vi "Process.vi"(0 "reference in":refnum<class "DCIR_HPPC.lvclass">, 5 "error in":errorcluster) -> (14 "reference out":refnum<class "DCIR_HPPC.lvclass">, 19 "error out":errorcluster)   [LabVIEW 2023, in "DCIR_HPPC.lvclass"]
uses:
  DCIR_HPPC.lvclass
  HPPC Parameters.ctl
  HPPC Mode.ctl
  Logger_class/Logger.lvclass
  builds/PowerModuleInterface/PowerModuleInterface.lvlibp/Classes/PowerModule_interface/PowerModuleInterface.lvclass
  <vilib>/Utility/NIReport.llb/Report Type.ctl
  <vilib>/printing/OpenHTMLReport.llb/Open HTML Report in Browser (Refnum).vi
  <vilib>/Utility/NIReport.llb/NI_report.lvclass
  DCIR_HPPC.lvclass/DCIR_HPPC.ctl
  <vilib>/Utility/SystemLogging/NI_SystemLogging.lvlib
  <userlib>/_OpenG.lib/time/time.llb/openg_time.lvlib
  <vilib>/Utility/NIReport.llb/NI_ReportGenerationCore.lvlib
panel:
  out "Last Command":string
  out "error info":errorcluster
  in  "Save HPPC Report":bool
  in  "HPPC Tab Control":T1(tab)
  out "HPPC Parameters":T2={"HPPC Mode"=1, "Pulse Duration (S)"=500.0, "Charge Current (A)"=1000.0, "Rest Duration (S)"=2.0, "Discharge Current (A)"=10.0, "Temperature (C)"=25.0, "Nominal Capacity (Ah)"=10.0, "Initial SoC (%)"=650.0, "Final SoC (%)"=50.0, "SoC Interval (%)"=10.0, "SoC Step Current (A)"=10.0, "SoC Step Relax (S)"=10.0} {"HPPC Mode" items=["One Shot (DCIR)", "Discharge Only", "Full Cycle"]; "Nominal Capacity (Ah)" min=0.0 max=100.0; "Final SoC (%)" min=0.0 max=100.0; "SoC Interval (%)" min=0.0 max=100.0; "Initial SoC (%)" min=0.0 max=100.0}
  out "HPPC Profile":waveform(dbl)[](graph)
  out "Running Status Log":i32(listbox) caption="TEST SERVER LOG"
  out "HPPC Step":dbl[][](graph)
  out "HPPC Voltage":cluster{dbl[], dbl[]}(graph)
  out "HPPC Power":cluster{dbl[], dbl[]}(graph)
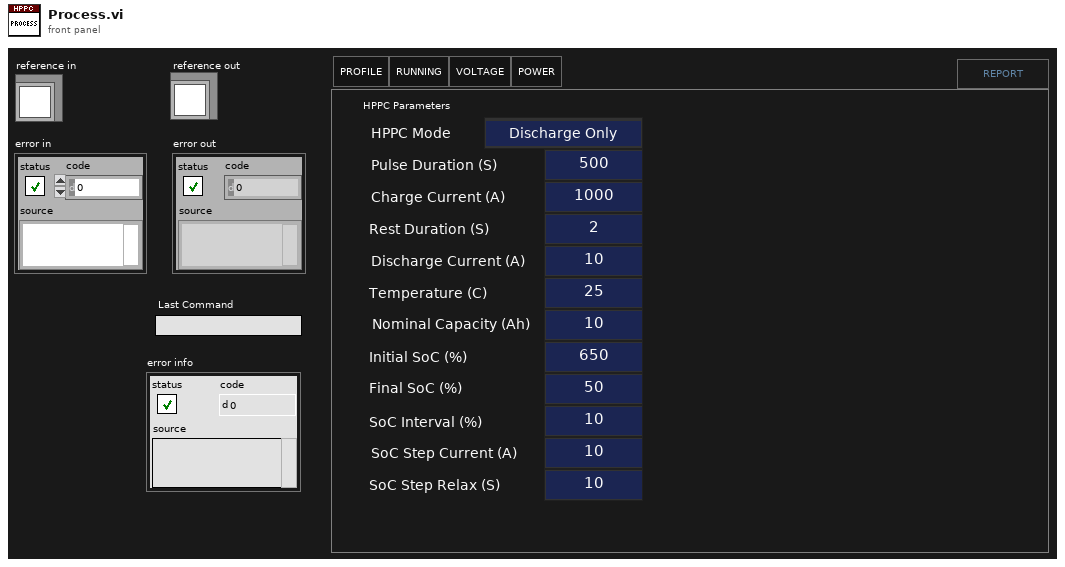
[diagram p1: front panel]
types:
  T1 = enum32{"PARAM", "PROFILE", "RUNNING", "VOLTAGE", "POWER"}
  T2 = typedef "DCIR_HPPC.lvclass/HPPC Parameters.ctl" = cluster{"HPPC Mode":T3, "Pulse Duration (S)":dbl, "Charge Current (A)":dbl, "Rest Duration (S)":dbl, "Discharge Current (A)":dbl, "Temperature (C)":dbl, "Nominal Capacity (Ah)":dbl, "Initial SoC (%)":dbl, "Final SoC (%)":dbl, "SoC Interval (%)":dbl, "SoC Step Current (A)":dbl, "SoC Step Relax (S)":dbl}
  T3 = typedef "DCIR_HPPC.lvclass/HPPC Mode.ctl" = u16
  T4 = cluster{"Core":cluster{"Timeout":i32, "Events":cluster{"EventsToProcess":refnum<event-registration>}, "EventFromProcess":refnum<user-event>, "ProcessSyncQueue":refnum<queue>, "QueueFromProcess":refnum<queue>, "Command":string, "Data":variant}, "HPPC Parameters":T2, "Profile Complete Event":refnum<user-event>, "HPPC Profile State":enum16{"Idle", "Start", "Run", "Stop"}, "HPPC TDMS Path":path, "Logger":refnum<class "Logger.lvclass">, "Power Module":refnum<class "PowerModuleInterface.lvclass">, "HPPC Profile":waveform(dbl), "HPPC States":cluster{"State":string, "Timestamp":dbl}[], "Last Timestamp (S)":dbl}
  T5 = enum8{"Enabled", "Disabled", "Disabled and Grayed Out"}
  T6 = typedef "NI_ReportGenerationCore.lvlib/Report Type.ctl" = enum16{"HTML", "Word", "Excel"}
  T7 = enum32{"Invalid", "Standard", "Closed", "Hidden", "Minimized", "Maximized"}
  T8 = cluster{"EventsToProcess":refnum<event-registration>}
  T9 = typedef "DCIR_HPPC.lvclass/ObjectAttributes.ctl" = cluster{"HPPC Parameters":T2, "Logger":refnum<class "Logger.lvclass">, "Power Module":refnum<class "PowerModuleInterface.lvclass">}
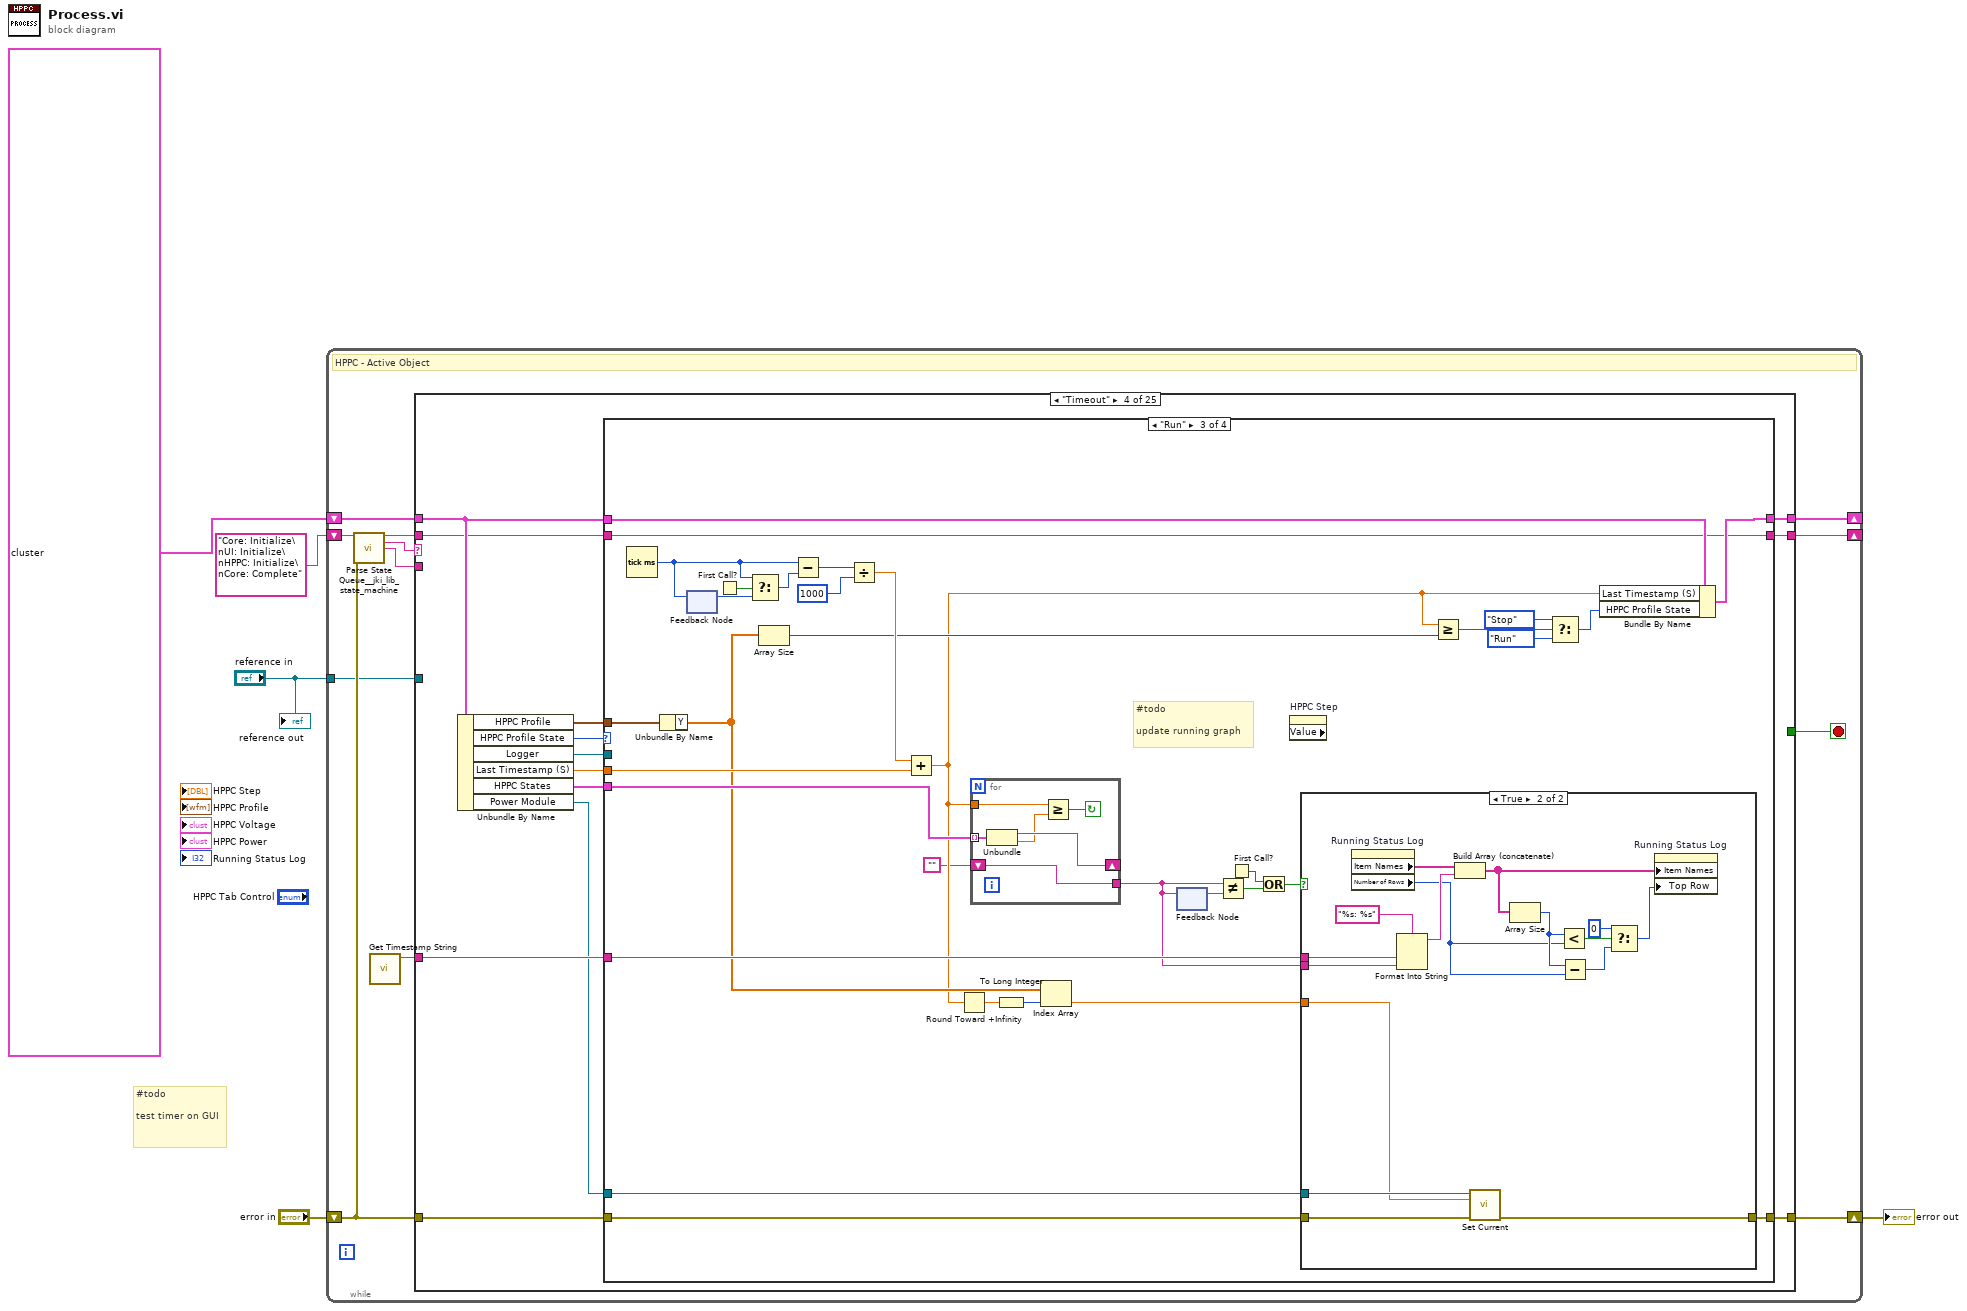
[diagram p0: block diagram]
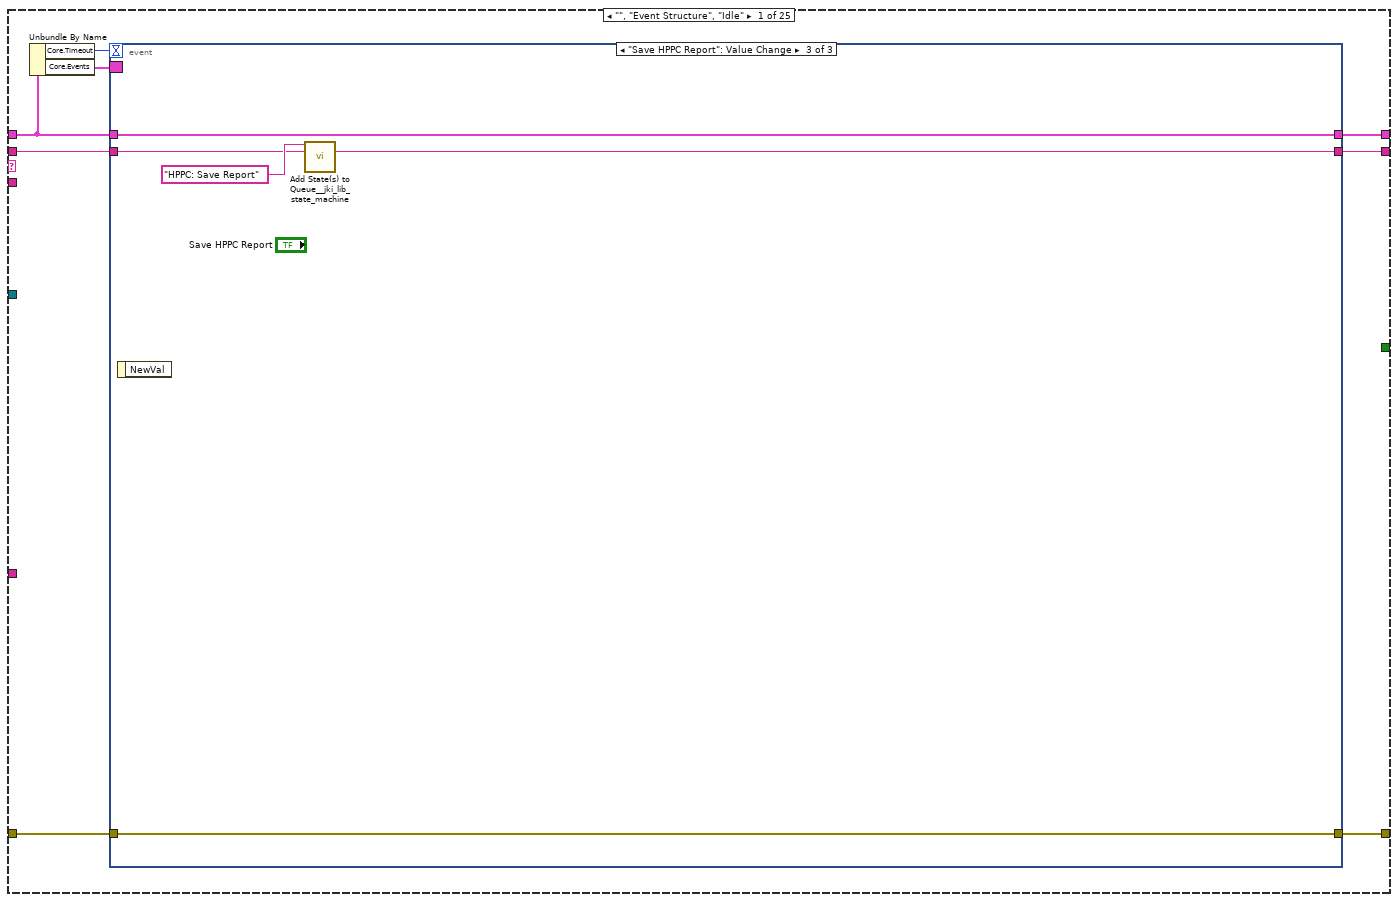
[diagram p2: hidden frame]
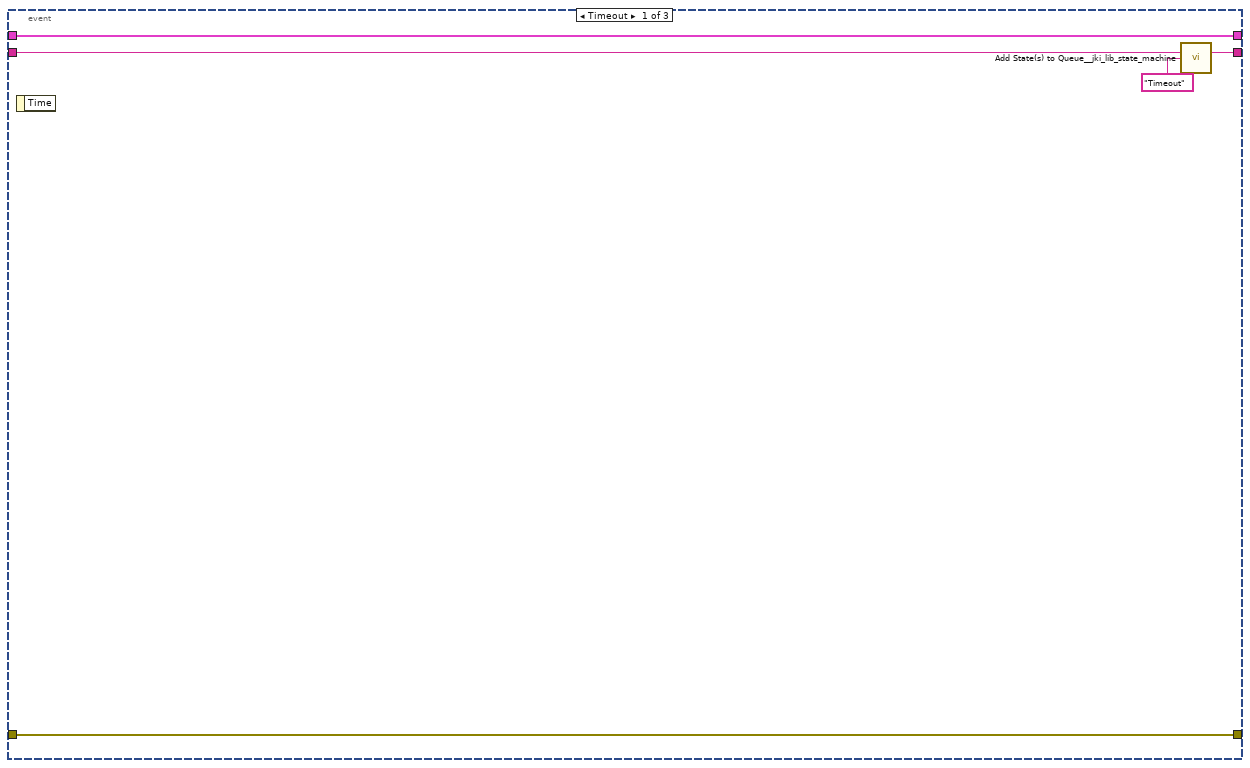
[diagram p3: hidden frame]
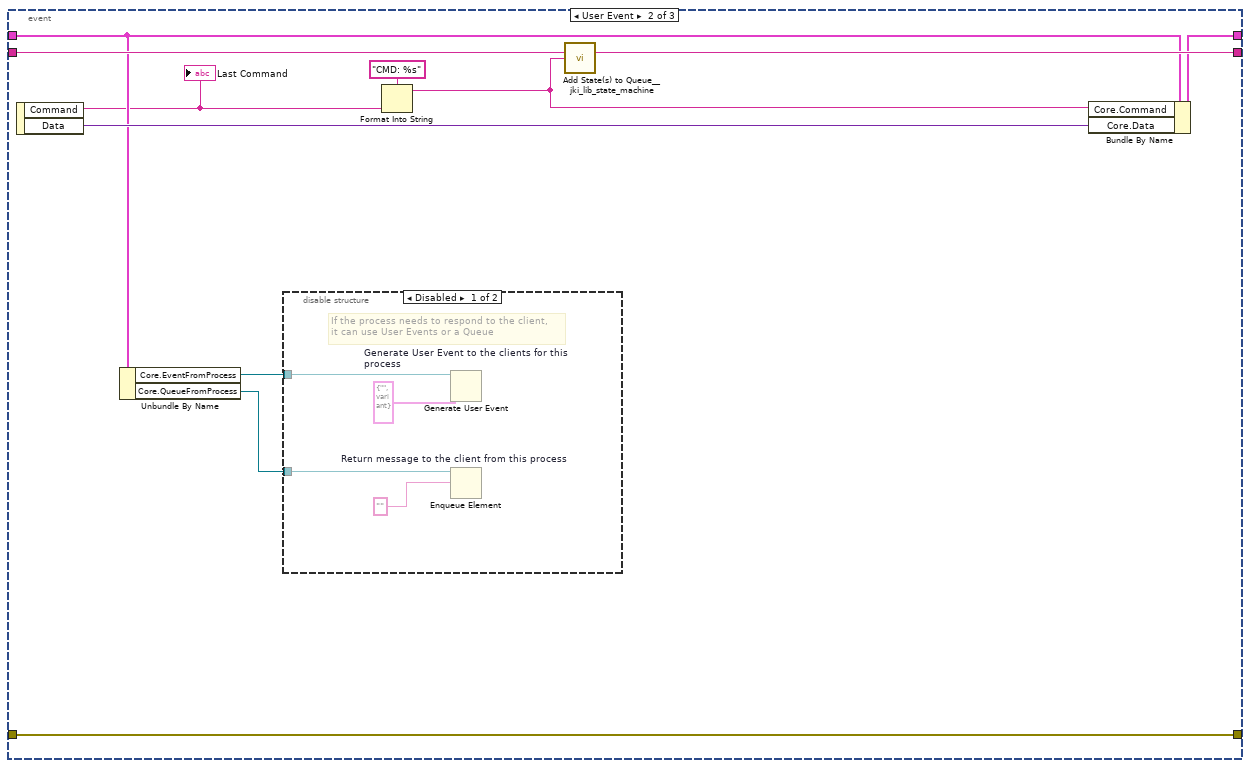
[diagram p4: hidden frame]
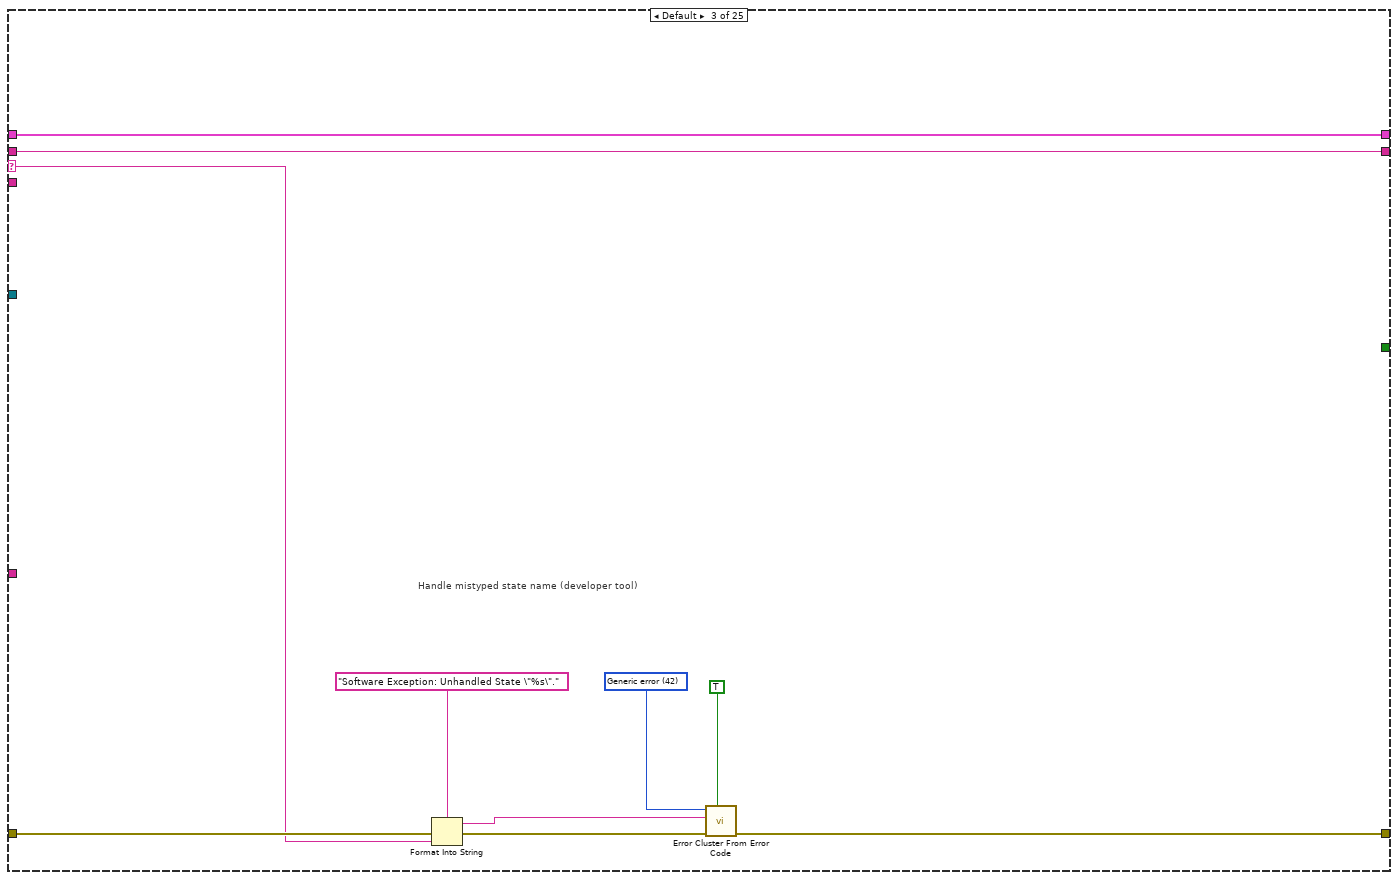
[diagram p7: hidden frame]
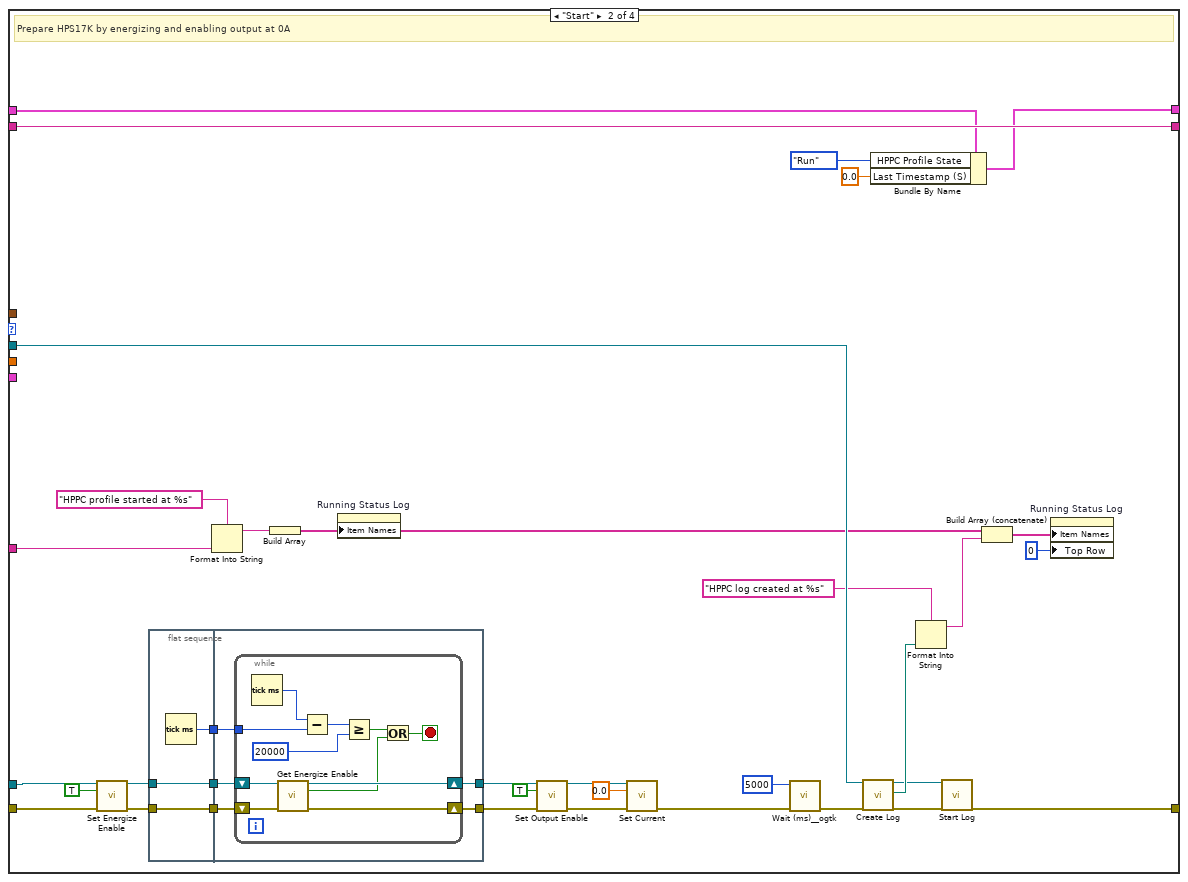
[diagram p9: hidden frame]
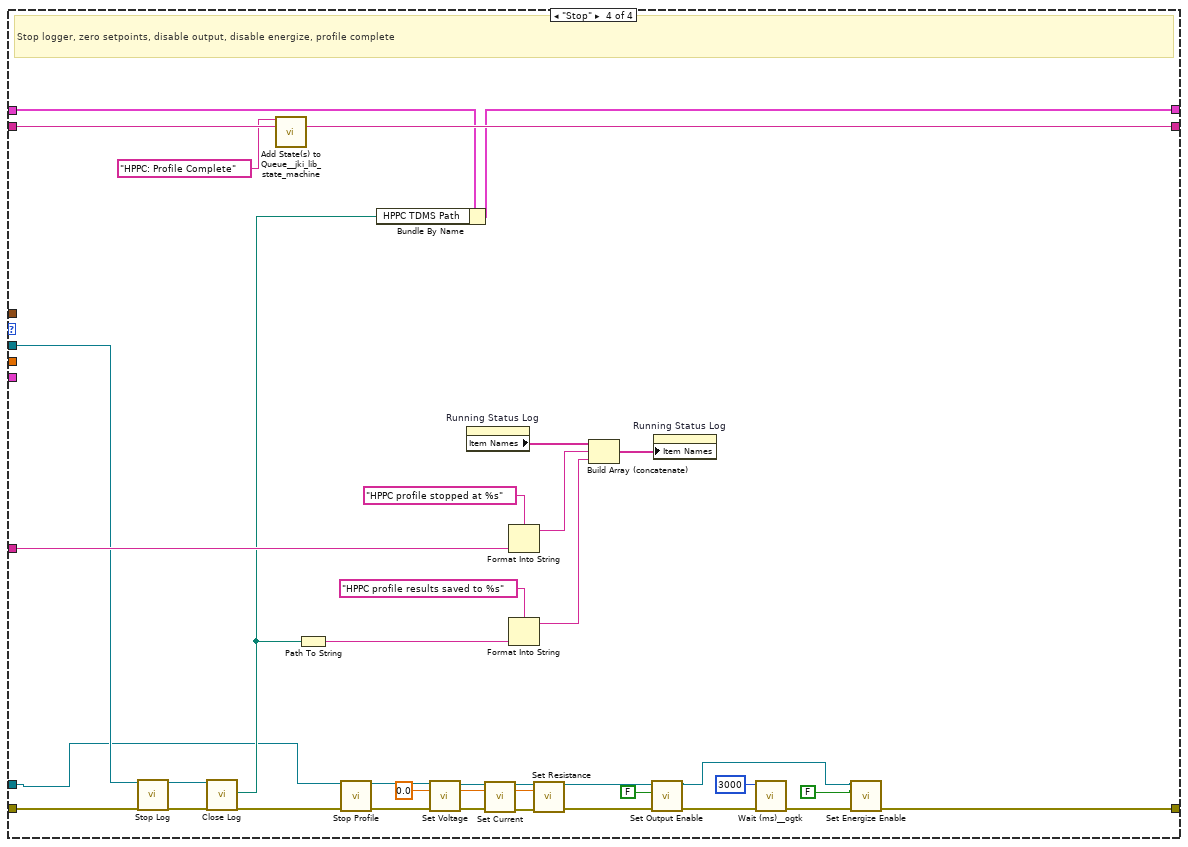
[diagram p11: hidden frame]
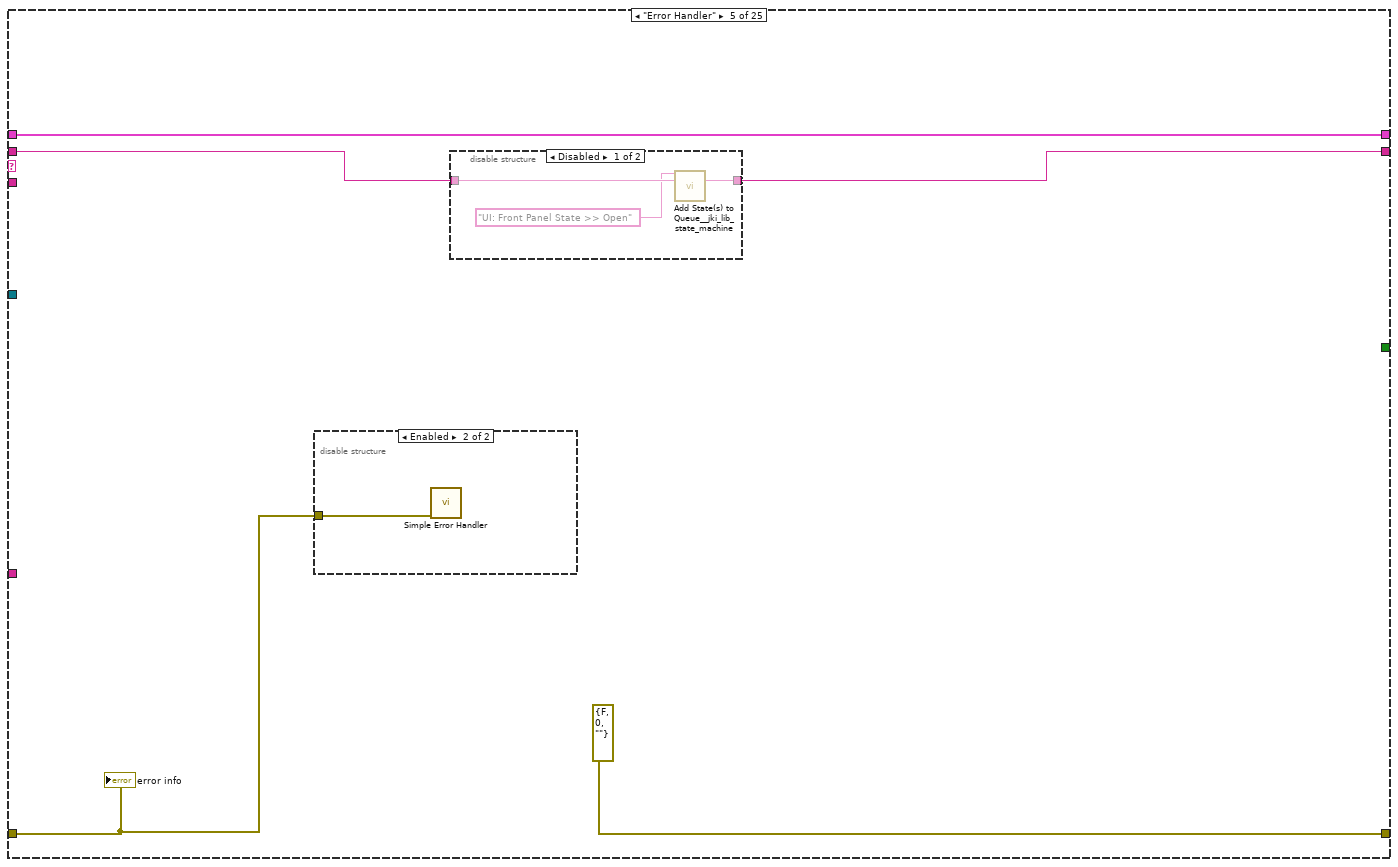
[diagram p12: hidden frame]
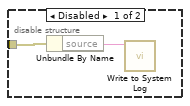
[diagram p14: hidden frame]
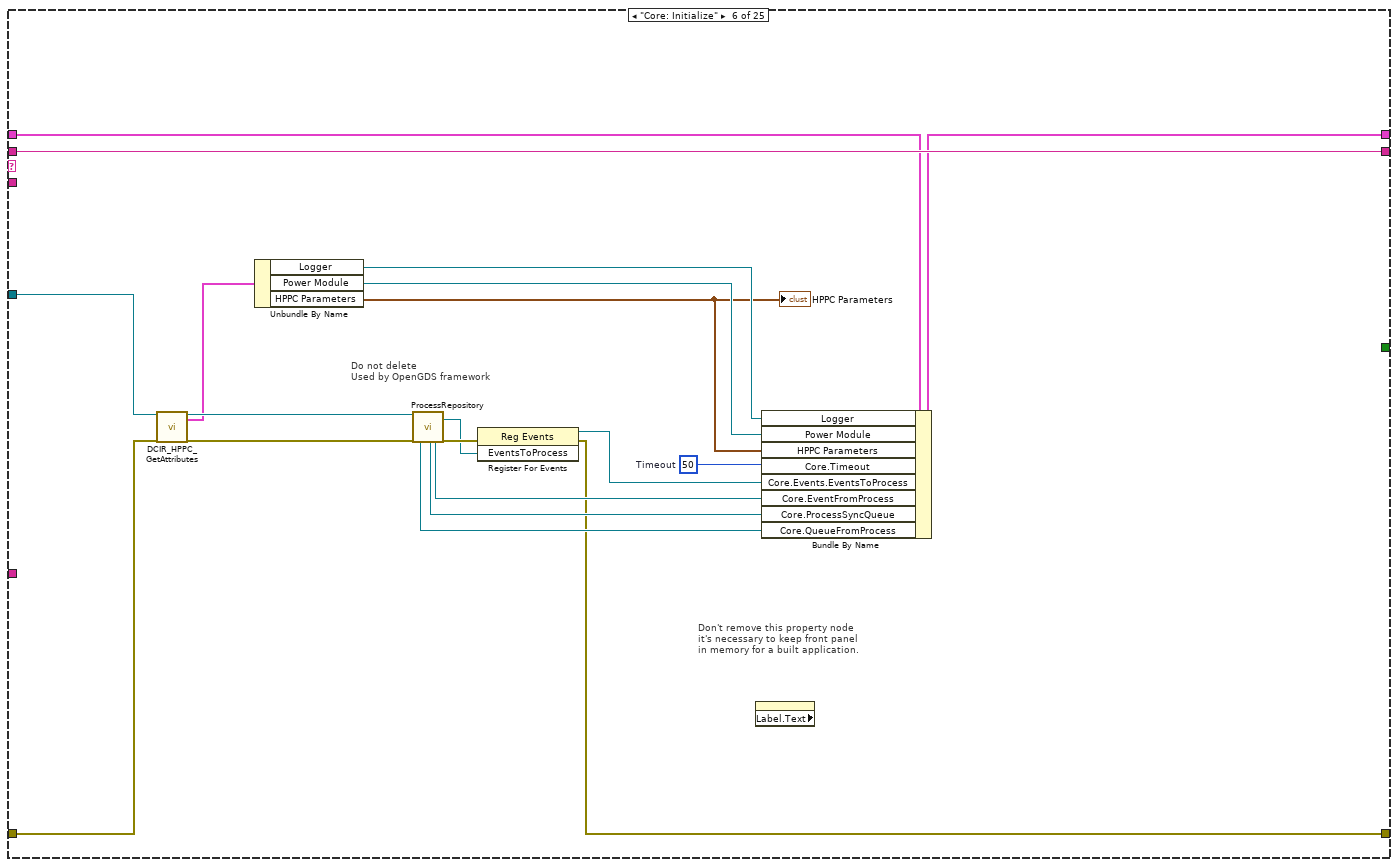
[diagram p15: hidden frame]
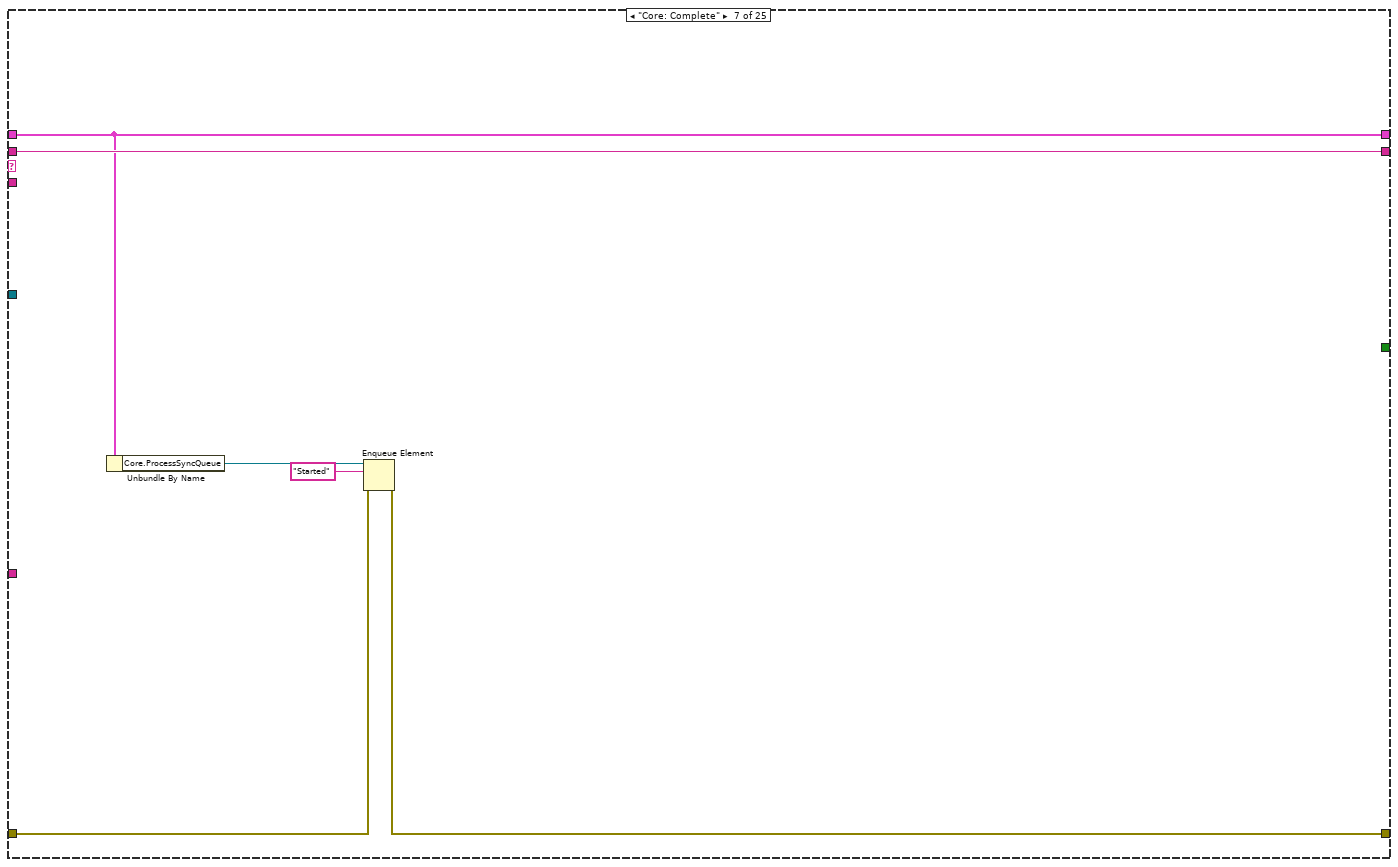
[diagram p16: hidden frame]
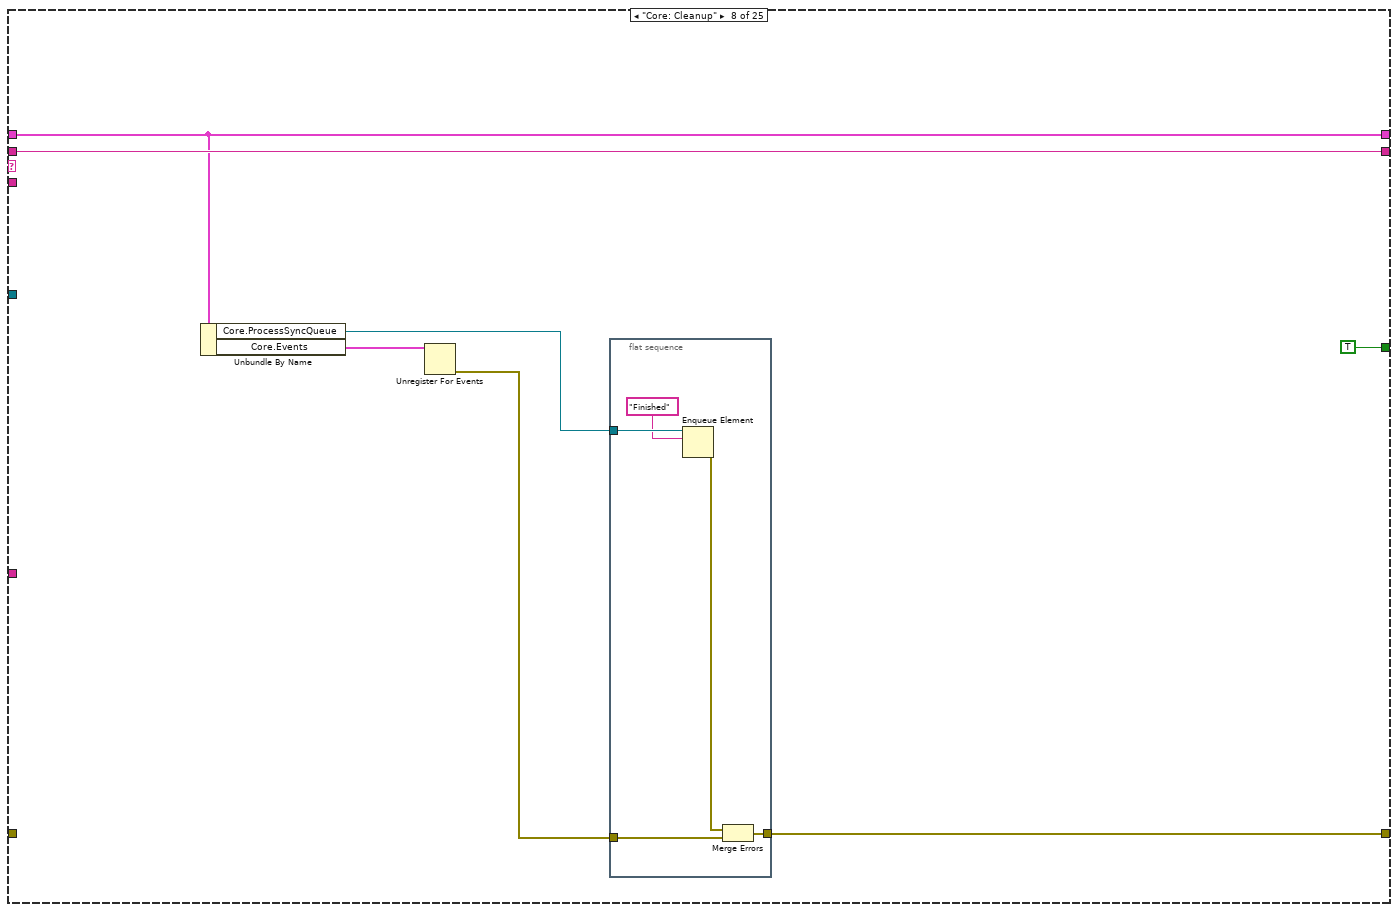
[diagram p17: hidden frame]
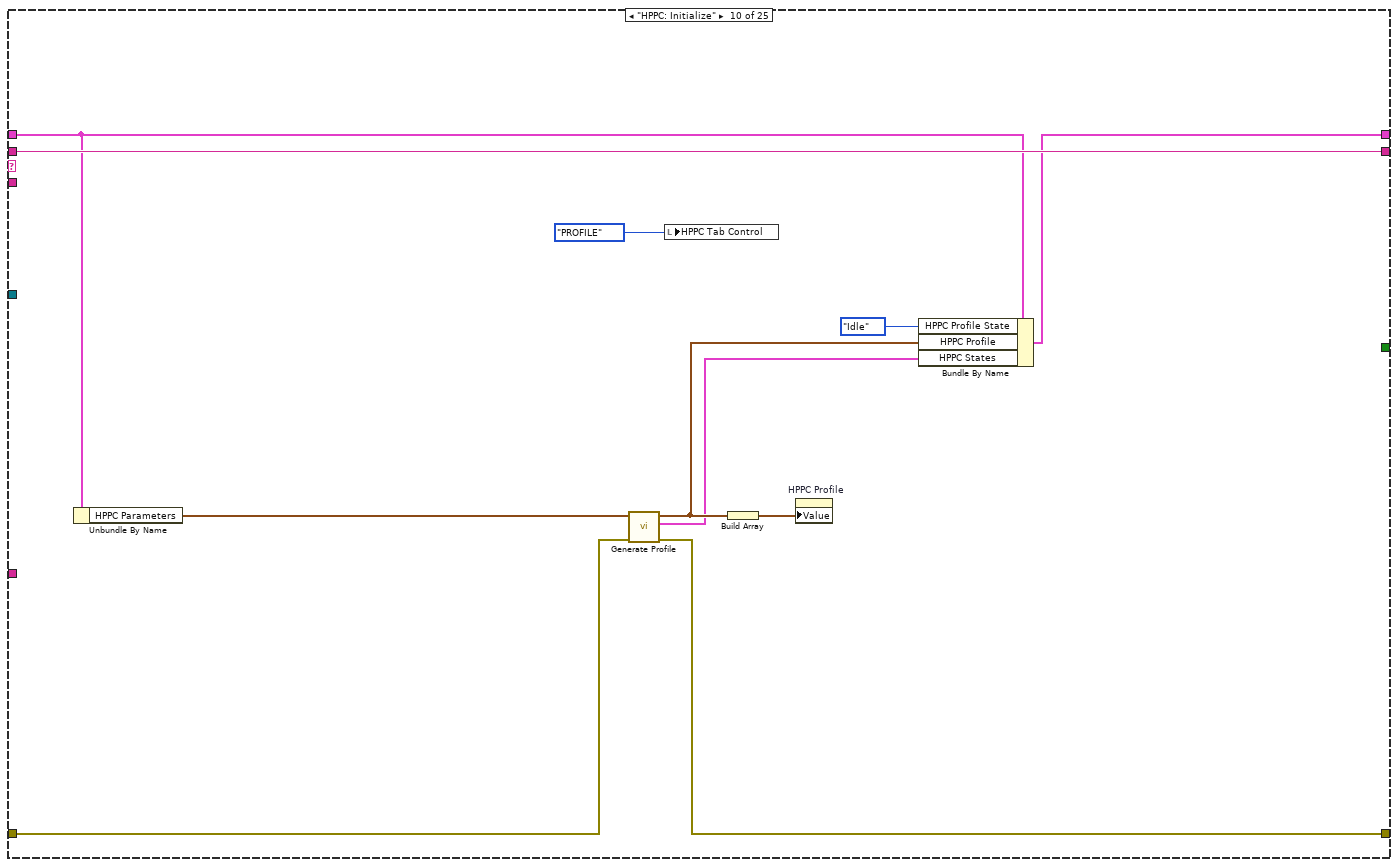
[diagram p19: hidden frame]
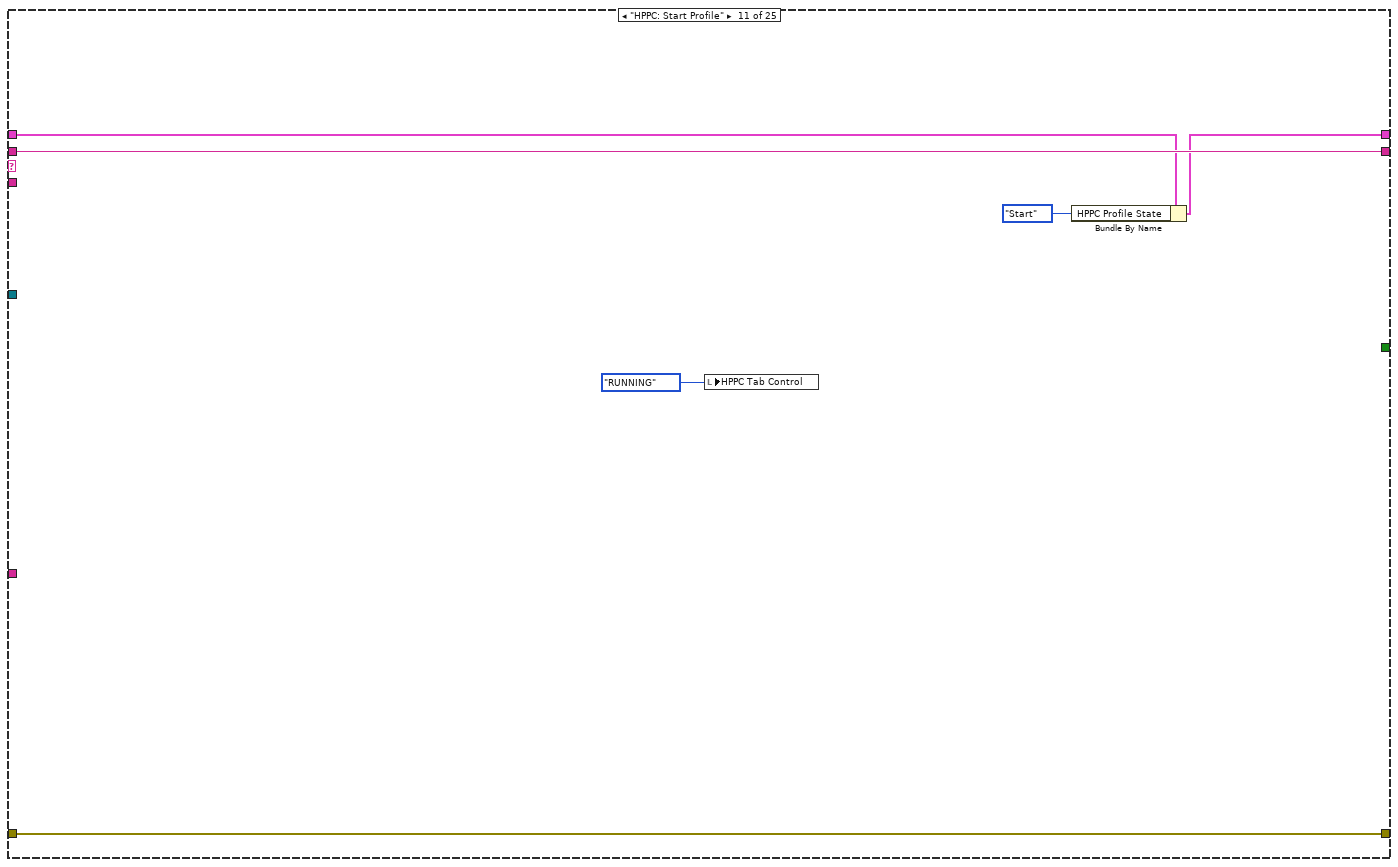
[diagram p20: hidden frame]
diagram:
  # "#todo\n\ntest timer on GUI"
  n1 = while {
    shift-right: [w16] -> w4
    shift-left: "error in" -> [w17]
    shift-right: [w9] -> _
    shift-left: "Core: Initialize\nUI: Initialize\nHPPC: Initialize\nCore: Complete" ("States Out") -> [w12]
    shift-right: [w15] -> _
    shift-left: T4 {"Core"={"Timeout"=-1, "Events"={"EventsToProcess"=refnum}, "EventFromProcess"=refnum, "ProcessSyncQueue"=refnum, "QueueFromProcess"=refnum, "Command"="", "Data"=variant}, "HPPC Parameters"={"HPPC Mode"=1, "Pulse Duration (S)"=500.0, "Charge Current (A)"=1000.0, "Rest Duration (S)"=2.0, "Discharge Current (A)"=10.0, "Temperature (C)"=25.0, "Nominal Capacity (Ah)"=10.0, "Initial SoC (%)"=650.0, "Final SoC (%)"=50.0, "SoC Interval (%)"=10.0, "SoC Step Current (A)"=10.0, "SoC Step Relax (S)"=10.0}, "Profile Complete Event"=refnum, "HPPC Profile State"=enum."Idle", "HPPC TDMS Path"=path "", "Logger"=refnum, "Power Module"=refnum, "HPPC Profile"={"t0"=timestamp(0 s since 1904-01-01), "dt"=1.0, "Y"=[]}, "HPPC States"=[], "Last Timestamp (S)"=0.0} ("LocalVariables") -> [w14]
    tunnel: "reference in" -> [w7]
    stop <- w8 stop-if-true
    # "HPPC - Active Object"
    n2 = call <vilib>:"Parse State Queue__jki_lib_state_machine.vi"("State Queue"=w12, "Error In (no error)"=w17) -> ("Remaining States"=w11:string, "Current State"=w13:string, "Arguments"=w10:string)  [unwired: 11 in]
    n3 = call "Get Timestamp String.vi"() -> ("date/time string"=w6:string)  [unwired: 11 in]
    n4 = case shown="\"Timeout\"" w13 {
      selector: w13 -> [_ _ w54 _ _ _ _ _ _ _ _ _ _ _ _ _ _ _ _ _ _ _ _ _ _]
      tunnel: w17 -> [w19 w53 w56 w76 w227 w242 w258 _ w277 w287 w294 w299 w306 w317 w323 w384 w385 w413 _ w420 w423 w430 w438 w445 w450]
      tunnel: [w20 w53 w55 w75 errorcluster {"status"=FALSE, "code"=0, "source"=""} ("error constant") w247 w262 w265 w277 w286 w294 w299 w305 w316 w321 w384 w385 w413 w414 w420 w423 w430 w437 w445 w450] -> w16
      tunnel: [w25 w52 w63 w71 w230 w255 w259 w266 w276 w285 w291 w296 w303 w319 w325 w383 w387 w412 w415 w419 w422 w429 w435 w444 w449] -> w15
      tunnel: w14 -> [w21 w52 w63 w72 w230 w254 w259 w266 w276 w283 w292 w297 w304 w319 w325 w383 w387 w412 w415 w419 w422 w429 w436 w444 w449]
      tunnel: w11 -> [w23 w51 w62 w70 w229 w256 w261 w269 w275 w288 w293 w298 w310 w320 w324 w382 w388 w396 w417 w418 _ w428 w433 w443 w447]
      tunnel: w10 -> [_ _ _ _ _ _ _ _ _ _ _ _ _ _ _ _ w386 _ _ _ _ w425 _ _ _]
      tunnel: [w22 w51 w62 w69 w228 w256 w261 w269 w275 w288 w293 w298 w310 w320 w324 w382 w388 w396 w417 w418 "UI: Cleanup\nCore: Cleanup" ("State(s) at Back (\"\")") w427 w432 w442 w446] -> w9
      tunnel: [_ _ _ _ _ _ _ TRUE _ _ _ _ _ _ _ _ _ _ _ _ _ _ _ _ _] -> w8
      tunnel: w7 -> [_ _ _ _ _ w245 _ _ _ _ _ _ _ _ _ _ _ _ _ _ _ _ _ _ _]
      tunnel: w6 -> [_ _ _ w73 _ _ _ _ _ _ _ _ _ _ w322 _ _ _ _ _ _ _ _ _ _]
      frame "", "Event Structure", "Idle" {
        n5 = Unbundle By Name(w21) -> ("Core.Timeout"=w18:i32, "Core.Events"=w24:T8)
        n6 = event shown="[2] \"Save HPPC Report\": Value Change" {
          selector: w24 -> [_ _ _]
          dyn-events: _ -> [_ _ _]
          timeout: w18 -> [_ _ _]
          tunnel: w21 -> [w30 w34 w50]
          tunnel: [w30 w39 w50] -> w25
          tunnel: [w28 w41 w46] -> w22
          tunnel: w23 -> [w29 w40 w47]
          tunnel: [w26 w35 w49] -> w20
          tunnel: w19 -> [w26 w35 w49]
          event Timeout {
            n7 = event-data() -> ()  [unwired: 1 in, 1 out]
            n8 = call <vilib>:"Add State(s) to Queue__jki_lib_state_machine.vi"("State(s) in (\"\")"=w29, "State(s) at Back (\"\")"="Timeout" ("State(s) at Back (\"\")")) -> ("States Out"=w28:string)  [unwired: 13 in]
          }
          event User Event {
            n9 = event-data() -> ("Command"=w32:string, "Data"=w38:variant)  [unwired: 1 in]
            "Last Command" <- w32
            n10 = Unbundle By Name(w34) -> ("Core.EventFromProcess"=w37:refnum<user-event>, "Core.QueueFromProcess"=w36:refnum<queue>)
            n11 = disable-structure shown="Disabled" {
              disable-tunnel: w37 -> [w45 _]
              disable-tunnel: w36 -> [w44 _]
              frame Disabled {
                # "If the process needs to respond to the client,\nit can use User Events or a Queue"
                n12 = Generate User Event "Generate User Event to the clients for this process"(user event=w45, event data cluster=cluster{"Command":string, "Data":variant} {"Command"="", "Data"=variant} ("event data")) -> ()  [unwired: 2 in, 2 out]
                n13 = Enqueue Element "Return message to the client from this process"(queue=w44, element="") -> ()  [unwired: 2 in, 3 out]
              }
              frame Enabled {
              }
            }
            n14 = Format Into String(format string="CMD: %s", w32) -> (resulting string=w31:string)  [unwired: 2 in, 1 out]
            n15 = call <vilib>:"Add State(s) to Queue__jki_lib_state_machine.vi"("State(s) in (\"\")"=w40, "State(s) at Back (\"\")"=w31) -> ("States Out"=w41:string)  [unwired: 13 in]
            n16 = Bundle By Name(cluster=w34, "Core.Command"=w31, "Core.Data"=w38) -> (w39:T4)
          }
          event "Save HPPC Report": Value Change {
            n17 = event-data() -> ()  [unwired: 1 in, 1 out]
            n18 = call <vilib>:"Add State(s) to Queue__jki_lib_state_machine.vi"("State(s) in Front (\"\")"="HPPC: Save Report" ("State(s) in Front (\"\")"), "State(s) in (\"\")"=w47) -> ("States Out"=w46:string)  [unwired: 13 in]
          }
        }
      }
      frame "---------- Core ----------" {
      }
      frame Default {
        w60 = 42 items=["No error", "Argument error", "Memory is full", "Out of zone", "End of file", "File already open", "Generic file I/O error", "File not found", "File permission error", "Disk is full", "Duplicate path", "Too many files open", "System feature not enabled", "Resource file not found", "Cannot add resource", "Resource not found", "Image not found", "Image memory error", "Pen does not exist", "Config type invalid", "Config token not found", "Config parse error", "Config memory error", "Bad external code format", "Bad external code offset", "External code not present", "Null window", "Destroy window error", "Null menu", "Print aborted", "Bad print record", "Print driver error", "Windows error during printing", "Memory error during printing", "Print dialog error", "Generic print error", "Invalid device refnum", "Device not found", "Device parameter error", "Device unit error", "Cannot open device", "Device call aborted", "Generic error", "Cancelled by user", "Object ID too low", "Object ID too high", "Object not in heap", "Unknown heap", "Unknown object (invalid DefProc)", "Unknown object (DefProc not in table)", "Message out of range", "Invalid (null) method", "Unknown message", "Manager call not supported", "Bad address", "Network operation in progress", "Network operation timed out", "Connection is busy", "Network attribute not supported", "Network error", "Address in use", "System out of memory", "Connection aborted", "Connection refused", "Not connected", "Already connected", "Connection closed", "Initialization error (interapplication manager)", "Bad occurrence", "Wait on unbound occurrence handler", "Occurrence queue overflow", "Datalog type conflict", "Unused", "Unrecognized type (interapplication manager)", "Memory corrupt", "Failed to make temporary DLL", "Old CIN version", "Drag socket not found", "Failed to load drop-object", "Failed to register OLE object", "Failed to release OLE object", "Format specifier type mismatch", "Unknown format specifier", "Too few format specifiers", "Too many format specifiers", "Scan failed", "Newer CIN version", "Error converting to variant", "Runtime menu error", "Password tampered", "Variant attribute not found", "Incompatible variant data type", "Event data is not available", "Event Store is not present", "Occurrence is not found", "Event Queue is not created", "Event info is not available", "Refnum passed is NULL", "Error retrieving Class GUID", "Error retrieving CoClass GUID", "Error retrieving TypeLib GUID.", "Bad built application magic bytes.", "Specific driver is different from the specific driver associated with the Logical Name.", "There is no session opened to the class driver.", "Max Error", "MAX - Error with config objects", "MAX - Error loading configuration", "MAX - Group not supported"]
        # "Handle mistyped state name (developer tool)"
        n19 = Format Into String(format string="Software Exception: Unhandled State \"%s\"." ("message"), error in=w56, w54) -> (resulting string=w59:string, error out=w58:errorcluster)  [unwired: 1 in]
        n20 = call <vilib>:"Error Cluster From Error Code.vi"("show call chain? (False)"=TRUE, "error in (no error)"=w58, "error message (\"\")"=w59, "error code (0)"=w60) -> ("error out"=w55:errorcluster)  [unwired: 5 in]
      }
      frame "Timeout" {
        n21 = Unbundle By Name(w72) -> ("HPPC Profile"=w67:waveform(dbl), "HPPC Profile State"=w74:enum16{"Idle", "Start", "Run", "Stop"}, "Logger"=w68:refnum<class "Logger.lvclass">, "Last Timestamp (S)"=w66:dbl, "HPPC States"=w64:cluster{"State":string, "Timestamp":dbl}[], "Power Module"=w65:refnum<class "PowerModuleInterface.lvclass">)
        n22 = case shown="\"Run\"" w74 {
          tunnel: w76 -> [w79 w85 w146 w217]
          tunnel: [w79 w103 w144 w191] -> w75
          tunnel: w65 -> [_ w83 w145 w190]
          tunnel: w68 -> [_ w114 _ w214]
          tunnel: w73 -> [_ w109 w147 w221]
          tunnel: w72 -> [w78 w101 w166 w213]
          tunnel: [w78 w100 w165 w212] -> w71
          tunnel: w70 -> [w77 w102 w164 w220]
          tunnel: [w77 w102 w164 w218] -> w69
          tunnel: w67 -> [_ _ w155 _]
          tunnel: w66 -> [_ _ w157 _]
          tunnel: w64 -> [_ _ w149 _]
          frame "Idle", Default {
            # "do nothing"
          }
          frame "Start" {
            # "Prepare HPS17K by energizing and enabling output at 0A"
            n23 = call-dynamic "Set Energize Enable.vi"("object in"=w83, "energize"=TRUE, "Error In"=w85) -> ("object out"=w93:refnum<class "PowerModuleInterface.lvclass">, "Error Out"=w92:errorcluster)  [unwired: 11 in]
            n24 = flat-sequence {
              tunnel: w93 -> [w116]
              tunnel: w92 -> [w117]
              tunnel: [w117] -> w96
              tunnel: [w116] -> w95
              tunnel: [w115] -> w94
              tunnel: [w120] -> w91
              tunnel: [w119] -> w90
              tunnel: w96 -> [w122]
              tunnel: w95 -> [w121]
              tunnel: w94 -> [w118]
              frame #0 {
                n25 = Tick Count (ms)() -> (millisecond timer value=w115:u32)
              }
              frame #1 {
                n26 = while {
                  shift-right: [w130] -> w119
                  shift-left: w122 -> [w133]
                  shift-right: [w131] -> w120
                  shift-left: w121 -> [w132]
                  tunnel: w118 -> [w126]
                  stop <- w128 stop-if-true
                  n27 = Tick Count (ms)() -> (millisecond timer value=w127:u32)
                  n28 = call-dynamic "Get Energize Enable.vi"("object in"=w132, "Error In"=w133) -> ("object out"=w131:refnum<class "PowerModuleInterface.lvclass">, "energized"=w129:bool, "Error Out"=w130:errorcluster)  [unwired: 11 in]
                  n29 = Subtract(x=w127, y=w126) -> (x-y=w125:u32)
                  n30 = Greater Or Equal?(x=w125, y=u32 20000 ("timeout (ms)")) -> (x >= y?=w123:bool)
                  n31 = Or(x=w123, y=w129) -> (x .or. y?=w128:bool)
                }
              }
            }
            n32 = Format Into String(format string="HPPC profile started at %s", w109) -> (resulting string=w98:string)  [unwired: 2 in, 1 out]
            n33 = Build Array(w98) -> (w97:string[])
            n34 = property on="Running Status Log" class="LstBox (strict)"("Item Names"=w97) -> ()  [unwired: 2 in, 2 out]
            n35 = call-dynamic "Set Output Enable.vi"("object in"=w91, "output"=TRUE, "Error In"=w90) -> ("object out"=w89:refnum<class "PowerModuleInterface.lvclass">, "Error Out"=w88:errorcluster)  [unwired: 11 in]
            n36 = call-dynamic "Set Current.vi"("object in"=w89, "current (A)"=0.0, "Error In"=w88) -> ("Error Out"=w82:errorcluster)  [unwired: 11 in, 1 out]
            n37 = call <userlib>:"Wait (ms)__ogtk.vi"("error in (no error)"=w82, "milliseconds to wait"=u32 5000) -> ("error out"=w113:errorcluster)  [unwired: 8 in, 1 out]
            n38 = call "Create Log.vi"("reference in"=w114, "Error In"=w113) -> ("reference out"=w106:refnum<class "Logger.lvclass">, "created file"=w107:path, "Error Out"=w111:errorcluster)  [unwired: 15 in]
            n39 = Bundle By Name(cluster=w101, "HPPC Profile State"=enum16{"Idle", "Start", "Run", "Stop"}."Run" ("EIS Profile State"), "Last Timestamp (S)"=0.0) -> (w100:T4)
            n40 = Format Into String(format string="HPPC log created at %s", w107) -> (resulting string=w105:string)  [unwired: 2 in, 1 out]
            n41 = call "Start Log.vi"("reference in"=w106, "Error In"=w111) -> ("Error Out"=w103:errorcluster)  [unwired: 16 in, 1 out]
            n42 = Build Array (concatenate)(w97, w105) -> (w104:string[])
            n43 = property on="Running Status Log" class="LstBox (strict)"("Item Names"=w104, "Top Row"=0) -> ()  [unwired: 2 in, 2 out]
          }
          frame "Run" {
            # "#todo\n\nupdate running graph"
            n44 = Tick Count (ms)() -> (millisecond timer value=w162:u32)
            n45 = Unbundle By Name(w155) -> ("Y"=w140:dbl[])
            n46 = feedback-in #1(w162) -> ()
            n47 = feedback #1() -> (w160:u32)  [unwired: 1 in]
            n48 = First Call?() -> (First Call?: T/F=w163:bool)
            n49 = Select(t=w162, s=w163, f=w160) -> (s? t:f=w161:u32)
            n50 = Array Size(array=w140) -> (size(s)=w154:i32)
            n51 = Subtract(x=w162, y=w161) -> (x-y=w159:u32)
            n52 = Divide(x=w159, y=u32 1000) -> (x/y=w156:dbl)
            n53 = Add(x=w156, y=w157) -> (x+y=w137:dbl)
            n54 = Round Toward +Infinity(x=w137) -> (ceil(x): smallest int >= x=w136:dbl)
            n55 = for {
              tunnel: w149 -> [w189] mode=indexing
              tunnel: w137 -> [w188]
              shift-right: [w187] -> _
              shift-left: "" -> [w184]
              tunnel: [w184] -> w134
              stop <- w185 continue-if-true
              n56 = Unbundle(w189) -> ("State"=w187:string, "Timestamp"=w186:dbl)
              n57 = Greater Or Equal?(x=w188, y=w186) -> (x >= y?=w185:bool)
            }
            n58 = To Long Integer(number=w136) -> (32bit integer=w139:i32)
            n59 = Index Array(array=w140, index=w139) -> (element=w138:dbl)
            n60 = feedback-in #2(w134) -> ()
            n61 = feedback #2() -> (w148:string)  [unwired: 1 in]
            n62 = Not Equal?(x=w134, y=w148) -> (x != y?=w143:bool)
            n63 = First Call?() -> (First Call?: T/F=w142:bool)
            n64 = Or(x=w142, y=w143) -> (x .or. y?=w141:bool)
            n65 = property on="HPPC Step" class="WFGraph (strict)" props=["Value"]() -> ()  [unwired: 2 in, 3 out]
            n66 = case shown="True" w141 {
              tunnel: w147 -> [_ w181]
              tunnel: w134 -> [_ w180]
              tunnel: w146 -> [w167 w178]
              tunnel: w145 -> [_ w177]
              tunnel: [w167 w176] -> w144
              tunnel: w138 -> [_ w175]
              frame False {
              }
              frame True {
                n67 = property on="Running Status Log" class="LstBox (strict)"() -> ("Item Names"=w183:string[], "Number of Rows"=w169:u32)  [unwired: 2 in, 2 out]
                n68 = Format Into String(format string="%s: %s", w181, w180) -> (resulting string=w179:string)  [unwired: 2 in, 1 out]
                n69 = Build Array (concatenate)(w183, w179) -> (w174:string[])
                n70 = call-dynamic "Set Current.vi"("object in"=w177, "current (A)"=w175, "Error In"=w178) -> ("Error Out"=w176:errorcluster)  [unwired: 11 in, 1 out]
                n71 = Array Size(array=w174) -> (size(s)=w170:i32)
                n72 = Less?(x=w170, y=w169) -> (x < y?=w173:bool)
                n73 = Subtract(x=w170, y=w169) -> (x-y=w168:u32)
                n74 = Select(t=0 ("size(s)"), s=w173, f=w168) -> (s? t:f=w171:u32)
                n75 = property on="Running Status Log" class="LstBox (strict)"("Item Names"=w174, "Top Row"=w171) -> ()  [unwired: 2 in, 2 out]
              }
            }
            n76 = Greater Or Equal?(x=w137, y=w154) -> (x >= y?=w153:bool)
            n77 = Select(t=enum16{"Idle", "Start", "Run", "Stop"}."Stop" ("HPPC Profile State"), s=w153, f=enum16{"Idle", "Start", "Run", "Stop"}."Run" ("HPPC Profile State")) -> (s? t:f=w151:enum16{"Idle", "Start", "Run", "Stop"})
            n78 = Bundle By Name(cluster=w166, "Last Timestamp (S)"=w137, "HPPC Profile State"=w151) -> (w165:T4)
          }
          frame "Stop" {
            w193 = 0.0 ("voltage (V)")
            # "Stop logger, zero setpoints, disable output, disable energize, profile complete"
            n79 = call "Stop Log.vi"("reference in"=w214, "Error In"=w217) -> ("reference out"=w215:refnum<class "Logger.lvclass">, "Error Out"=w216:errorcluster)  [unwired: 16 in]
            n80 = call "Close Log.vi"("reference in"=w215, "Error In"=w216) -> ("log file path"=w208:path, "Error Out"=w192:errorcluster)  [unwired: 15 in, 1 out]
            n81 = call <vilib>:"Add State(s) to Queue__jki_lib_state_machine.vi"("State(s) in Front (\"\")"="HPPC: Profile Complete" ("State(s) in Front (\"\")"), "State(s) in (\"\")"=w220) -> ("States Out"=w218:string)  [unwired: 13 in]
            n82 = Path To String(path=w208) -> (string=w210:string)
            n83 = call-dynamic "Stop Profile.vi"("object in"=w190, "Error In"=w192) -> ("object out"=w194:refnum<class "PowerModuleInterface.lvclass">, "Error Out"=w201:errorcluster)  [unwired: 12 in]
            n84 = Bundle By Name(cluster=w213, "HPPC TDMS Path"=w208) -> (w212:T4)
            n85 = call-dynamic "Set Voltage.vi"("object in"=w194, "voltage (V)"=w193, "Error In"=w201) -> ("object out"=w195:refnum<class "PowerModuleInterface.lvclass">, "Error Out"=w200:errorcluster)  [unwired: 11 in]
            n86 = property on="Running Status Log" class="LstBox (strict)"() -> ("Item Names"=w225:string[])  [unwired: 2 in, 2 out]
            n87 = call-dynamic "Set Current.vi"("object in"=w195, "current (A)"=w193, "Error In"=w200) -> ("object out"=w196:refnum<class "PowerModuleInterface.lvclass">, "Error Out"=w199:errorcluster)  [unwired: 11 in]
            n88 = Format Into String(format string="HPPC profile stopped at %s", w221) -> (resulting string=w224:string)  [unwired: 2 in, 1 out]
            n89 = Format Into String(format string="HPPC profile results saved to %s", w210) -> (resulting string=w209:string)  [unwired: 2 in, 1 out]
            n90 = call-dynamic "Set Resistance.vi"("object in"=w196, "resistance (Ohm)"=w193, "Error In"=w199) -> ("object out"=w197:refnum<class "PowerModuleInterface.lvclass">, "Error Out"=w198:errorcluster)  [unwired: 11 in]
            n91 = Build Array (concatenate)(w225, w224, w209) -> (w223:string[])
            n92 = call-dynamic "Set Output Enable.vi"("object in"=w197, "output"=FALSE ("enabled output"), "Error In"=w198) -> ("object out"=w203:refnum<class "PowerModuleInterface.lvclass">, "Error Out"=w204:errorcluster)  [unwired: 11 in]
            n93 = property on="Running Status Log" class="LstBox (strict)"("Item Names"=w223) -> ()  [unwired: 2 in, 2 out]
            n94 = call <userlib>:"Wait (ms)__ogtk.vi"("error in (no error)"=w204, "milliseconds to wait"=u32 3000) -> ("error out"=w206:errorcluster)  [unwired: 8 in, 1 out]
            n95 = call-dynamic "Set Energize Enable.vi"("object in"=w203, "energize"=FALSE ("energize (T)"), "Error In"=w206) -> ("Error Out"=w191:errorcluster)  [unwired: 11 in, 1 out]
          }
        }
      }
      frame "Error Handler" {
        n96 = disable-structure shown="Enabled" {
          disable-tunnel: w227 -> [w236 w237]
          frame Disabled {
            n97 = Unbundle By Name(w236) -> ("source"=w235:string)
            n98 = call <vilib>:"Write to System Log.vi"("message"=w235) -> ()  [unwired: 10 in, 1 out]
          }
          frame Enabled {
            n99 = call <vilib>:"Simple Error Handler.vi"("error in (no error)"=w237) -> ()  [unwired: 4 in, 5 out]
          }
        }
        n100 = disable-structure shown="Disabled" {
          disable-tunnel: w229 -> [w233 w234]
          disable-tunnel: [w232 w234] -> w228
          frame Disabled {
            n101 = call <vilib>:"Add State(s) to Queue__jki_lib_state_machine.vi"("State(s) in Front (\"\")"="UI: Front Panel State >> Open" ("State(s) at Back (\"\")"), "State(s) in (\"\")"=w233) -> ("States Out"=w232:string)  [unwired: 13 in]
          }
          frame Enabled {
          }
        }
        "error info" <- w227
      }
      frame "Core: Initialize" {
        w246 = 50  # Timeout
        # "Do not delete\nUsed by OpenGDS framework"
        # "Don't remove this property node\nit's necessary to keep front panel\nin memory for a built application."
        # "Template created by VI Technologies"
        n102 = call "DCIR_HPPC_GetAttributes.vi"("reference in"=w245, "Error In"=w242) -> ("reference out"=w244:refnum<class "DCIR_HPPC.lvclass">, "Data"=w241:T9, "Error Out"=w243:errorcluster)  [unwired: 14 in, 1 out]
        n103 = Unbundle By Name(w241) -> ("Logger"=w239:refnum<class "Logger.lvclass">, "Power Module"=w240:refnum<class "PowerModuleInterface.lvclass">, "HPPC Parameters"=w238:T2)
        "HPPC Parameters" <- w238
        n104 = call "ProcessRepository.vi"("reference in"=w244, "Error In"=w243) -> ("QueueFromProcess"=w249:refnum<queue>, "ProcessSyncQueue"=w248:refnum<queue>, "EventFromProcess"=w250:refnum<user-event>, "EventsToProcess"=w252:refnum<user-event>, "Error Out"=w253:errorcluster)  [unwired: 10 in, 3 out]
        n105 = register-events(error in=w253, w252) -> (reference out=w251:refnum<event-registration>, error out=w247:errorcluster)  [unwired: 1 in]
        n106 = property on="reference in" class="LVClassControl (strict)" props=["Label", "Text"]() -> ()  [unwired: 2 in, 3 out]
        n107 = Bundle By Name(cluster=w254, "Logger"=w239, "Power Module"=w240, "HPPC Parameters"=w238, "Core.Timeout"=w246, "Core.Events.EventsToProcess"=w251, "Core.EventFromProcess"=w250, "Core.ProcessSyncQueue"=w248, "Core.QueueFromProcess"=w249) -> (w255:T4)
      }
      frame "Core: Complete" {
        # "Template created by VI Technologies"
        n108 = Unbundle By Name(w259) -> ("Core.ProcessSyncQueue"=w257:refnum<queue>)
        n109 = Enqueue Element(queue=w257, element="Started", error in (no error)=w258) -> (error out=w262:errorcluster)  [unwired: 1 in, 2 out]
      }
      frame "Core: Cleanup" {
        n110 = Unbundle By Name(w266) -> ("Core.ProcessSyncQueue"=w267:refnum<queue>, "Core.Events"=w264:T8)
        n111 = Unregister For Events(event registration refnum=w264) -> (error out=w263:errorcluster)  [unwired: 1 in]
        n112 = flat-sequence {
          tunnel: [w273] -> w265
          tunnel: w267 -> [w272]
          tunnel: w263 -> [w271]
          frame #0 {
            n113 = Enqueue Element(queue=w272, element="Finished") -> (error out=w274:errorcluster)  [unwired: 2 in, 2 out]
            n114 = Merge Errors(w274, w271) -> (w273:errorcluster)
          }
        }
      }
      frame "---------- HPPC ----------" {
      }
      frame "HPPC: Initialize" {
        n115 = Unbundle By Name(w283) -> ("HPPC Parameters"=w280:T2)
        n116 = call "Generate Profile.vi"("error in (no error)"=w287, "HPPC Parameters"=w280) -> ("error out"=w286:errorcluster, "HPPC States"=w278:cluster{"State":string, "Timestamp":dbl}[], "HPPC Profile"=w282:waveform(dbl))  [unwired: 7 in]
        n117 = local write "HPPC Tab Control"(T1."PROFILE" ("DCIR Tab Control")) -> ()
        n118 = Build Array(w282) -> (w281:waveform(dbl)[])
        n119 = property on="HPPC Profile" class="WFGraph (strict)"("Value"=w281) -> ()  [unwired: 2 in, 2 out]
        n120 = Bundle By Name(cluster=w283, "HPPC Profile State"=enum16{"Idle", "Start", "Run", "Stop"}."Idle" ("EIS Profile State"), "HPPC Profile"=w282, "HPPC States"=w278) -> (w285:T4)
      }
      frame "HPPC: Start Profile" {
        n121 = local write "HPPC Tab Control"(T1."RUNNING" ("DCIR Tab Control")) -> ()
        n122 = Bundle By Name(cluster=w292, "HPPC Profile State"=enum16{"Idle", "Start", "Run", "Stop"}."Start" ("EIS Profile State")) -> (w291:T4)
      }
      frame "HPPC: Stop Profile" {
        n123 = Bundle By Name(cluster=w297, "HPPC Profile State"=enum16{"Idle", "Start", "Run", "Stop"}."Stop" ("EIS Profile State")) -> (w296:T4)
      }
      frame "HPPC: Profile Complete" {
        n124 = Unbundle By Name(w304) -> ("Profile Complete Event"=w309:refnum<user-event>, "HPPC TDMS Path"=w302:path)
        n125 = Path To String(path=w302) -> (string=w301:string)
        n126 = Format Into String(format string="HPPC Profile data saved to %s" ("event data"), w301) -> (resulting string=w307:string)  [unwired: 2 in, 1 out]
        n127 = Generate User Event(user event=w309, event data cluster=w307, error in=w306) -> (error out=w305:errorcluster)  [unwired: 1 in, 1 out]
        n128 = Bundle By Name(cluster=w304, "HPPC Profile State"=enum16{"Idle", "Start", "Run", "Stop"}."Idle" ("EIS Profile State")) -> (w303:T4)
      }
      frame "HPPC: Generate Plots" {
        n129 = Unbundle By Name(w319) -> ("HPPC TDMS Path"=w318:path, "HPPC Parameters"=w314:T2)
        n130 = call "Generate HPPC Plots.vi"("error in (no error)"=w317, "HPPC Parameters"=w314, "TDMS Data File"=w318) -> ("error out"=w316:errorcluster, "HPPC Power"=w311:cluster{dbl[], dbl[]}, "HPPC Voltage"=w312:cluster{dbl[], dbl[]})  [unwired: 6 in]
        n131 = local write "HPPC Tab Control"(T1."VOLTAGE" ("DCIR Tab Control")) -> ()
        n132 = property on="Save HPPC Report" class="Bool"("DisabledEnum"=T5."Enabled" ("Disabled")) -> ()  [unwired: 2 in, 2 out]
        n133 = local write "HPPC Power"(w311) -> ()
        n134 = local write "HPPC Voltage"(w312) -> ()
      }
      frame "HPPC: Save Report" {
        n135 = disable-structure shown="TARGET_TYPE==Windows, Default" {
          disable-tunnel: w323 -> [w334 w381]
          disable-tunnel: w322 -> [w328 _]
          disable-tunnel: [w326 w381] -> w321
          frame condition #0 (active) {
            n136 = call "File Dialog"("error in"=w334, "pattern (all files)"="*.html", "pattern label"="HTML Report") -> ("selected path"=w327:path, "cancelled"=w331:bool, "error out"=w329:errorcluster)  [unwired: 9 in, 1 out]
            n137 = Or(x=w331, y=w329) -> (x .or. y?=w330:bool)
            n138 = case shown="False" w330 {
              tunnel: w329 -> [w378 w380]
              tunnel: w328 -> [w373 _]
              tunnel: w327 -> [w370 _]
              tunnel: [w365 w380] -> w326
              frame False {
                w336 = enum16{".jpg", ".png"}.".png" ("image file type (.jpg)")
                n139 = call <vilib>:"Create Report.vi"("report type"=Report_Type."HTML", "error in (no error)"=w378) -> ("report out"=w376:refnum<class "NI_report.lvclass">, "error out"=w377:errorcluster)  [unwired: 12 in]
                n140 = property on="Running Status Log" class="LstBox (strict)"() -> ("Item Names"=w368:string[])  [unwired: 2 in, 2 out]
                n141 = call-dynamic "Set Report Header Text.vi"("report in"=w376, "left header text"="Volta Control Suite", "center header text"="HPPC Report", "right header text"=w373, "error in (no error)"=w377) -> ("report out"=w356:refnum<class "NI_report.lvclass">, "error out"=w357:errorcluster)  [unwired: 9 in]
                n142 = call-dynamic "Append Horizontal Line to Report.vi"("report in"=w356, "error in (no error)"=w357) -> ("report out"=w354:refnum<class "NI_report.lvclass">, "error out"=w355:errorcluster)  [unwired: 12 in]
                n143 = control-ref of="HPPC Profile"() -> (w364:refnum<vi>)
                n144 = call-dynamic "Append List to Report.vi"("report in"=w354, "list elements"=w368, "error in (no error)"=w355) -> ("report out"=w352:refnum<class "NI_report.lvclass">, "error out"=w353:errorcluster)  [unwired: 9 in, 2 out]
                n145 = control-ref of="HPPC Power"() -> (w335:refnum<vi>)
                n146 = control-ref of="HPPC Voltage"() -> (w371:refnum<vi>)
                n147 = control-ref of="HPPC Parameters"() -> (w358:refnum<vi>)
                n148 = call-dynamic "Append Horizontal Line to Report.vi"("report in"=w352, "error in (no error)"=w353) -> ("report out"=w350:refnum<class "NI_report.lvclass">, "error out"=w351:errorcluster)  [unwired: 12 in]
                n149 = call-dynamic "Append Control Image to Report.vi"("report in"=w350, "ctrl reference"=w358, "description"="HPPC Parameters", "error in (no error)"=w351) -> ("report out"=w348:refnum<class "NI_report.lvclass">, "error out"=w349:errorcluster)  [unwired: 8 in, 2 out]
                n150 = call-dynamic "Append Horizontal Line to Report.vi"("report in"=w348, "error in (no error)"=w349) -> ("report out"=w346:refnum<class "NI_report.lvclass">, "error out"=w347:errorcluster)  [unwired: 12 in]
                n151 = call-dynamic "Append Control Image to Report.vi"("report in"=w346, "image file type (.jpg)"=w336, "ctrl reference"=w364, "description"="HPPC Profile", "error in (no error)"=w347) -> ("report out"=w344:refnum<class "NI_report.lvclass">, "error out"=w345:errorcluster)  [unwired: 7 in, 2 out]
                n152 = call-dynamic "Append Horizontal Line to Report.vi"("report in"=w344, "error in (no error)"=w345) -> ("report out"=w342:refnum<class "NI_report.lvclass">, "error out"=w343:errorcluster)  [unwired: 12 in]
                n153 = call-dynamic "Append Control Image to Report.vi"("report in"=w342, "image file type (.jpg)"=w336, "ctrl reference"=w371, "description"="HPPC Voltage", "error in (no error)"=w343) -> ("report out"=w337:refnum<class "NI_report.lvclass">, "error out"=w340:errorcluster)  [unwired: 7 in, 2 out]
                n154 = call-dynamic "Append Control Image to Report.vi"("report in"=w337, "image file type (.jpg)"=w336, "ctrl reference"=w335, "description"="HPPC Power", "error in (no error)"=w340) -> ("report out"=w338:refnum<class "NI_report.lvclass">, "error out"=w339:errorcluster)  [unwired: 7 in, 2 out]
                n155 = call-dynamic "Append User Formatted HTML to Report.vi"("report in"=w338, "HTML text"="<style>body {background-color:#111111;color:#ECECED}</style>", "error in (no error)"=w339) -> ("report out"=w362:refnum<class "NI_report.lvclass">, "error out"=w363:errorcluster)  [unwired: 11 in]
                n156 = call-dynamic "Save Report to File.vi"("report in"=w362, "report file path"=w370, "prompt to replace? (F)"=TRUE, "error in (no error)"=w363) -> ("report out"=w367:refnum<class "NI_report.lvclass">, "error out"=w366:errorcluster)  [unwired: 10 in]
                n157 = call-poly <vilib>:"Open HTML Report in Browser.vi"("report in"=w367, "error in (no error)"=w366) -> ("error out"=w365:errorcluster)  [unwired: 11 in, 2 out]
              }
              frame True {
              }
            }
          }
          frame condition #1 {
          }
        }
      }
      frame "---------- UI ----------" {
      }
      frame "UI: Front Panel State" {
        n158 = case shown="\"Close\"" w386 {
          frame "Open", Default {
            n159 = property class="VI"() -> ("FP.State"=w389:T7)  [unwired: 2 in, 2 out]
            n160 = case shown="Default" w389 {
              frame Default {
                n161 = invoke class="VI" method="FP.Open"("Activate"=TRUE, "State"=T7."Standard") -> ()  [unwired: 3 in, 5 out]
              }
              frame "Standard" {
              }
            }
          }
          frame "Close" {
            n162 = property class="VI"() -> ("FP.State"=w392:T7)  [unwired: 2 in, 2 out]
            n163 = case shown="Default" w392 {
              frame "Closed" {
              }
              frame Default {
                n164 = invoke class="VI" method="FP.Close"() -> ()  [unwired: 3 in, 3 out]
              }
            }
          }
        }
      }
      frame "UI: Initialize" {
        n165 = property class="VI"() -> ("Name"=w409:string)  [unwired: 2 in, 2 out]
        n166 = Match Pattern(string=w409, regular expression="\\2Evi$") -> (before substring=w407:string)  [unwired: 1 in, 3 out]
        n167 = local write "HPPC Tab Control"(T1."PROFILE" ("DCIR Tab Control")) -> ()
        n168 = property on="Running Status Log" class="LstBox (strict)"("Item Names"=string[] []) -> ()  [unwired: 2 in, 2 out]
        n169 = Reverse String(1:w407) -> (0:w406:string)
        n170 = Match Pattern(string=w406, regular expression=":") -> (before substring=w404:string, after substring=w403:string)  [unwired: 1 in, 2 out]
        n171 = local write "HPPC Voltage"(cluster{dbl[], dbl[]} {[], []} ("EIS Nyquist")) -> ()
        n172 = local write "HPPC Profile"(waveform(dbl)[] [] ("EIS Profile")) -> ()
        n173 = Match Pattern(string=w403, regular expression="\\2E") -> (after substring=w401:string)  [unwired: 1 in, 3 out]
        n174 = Reverse String(1:w401) -> (0:w400:string)
        n175 = Reverse String(1:w404) -> (0:w399:string)
        n176 = Format Into String(format string="%s %s", w400, w399) -> (resulting string=w398:string)  [unwired: 2 in, 1 out]
        n177 = property class="VI"("Front Panel.Title"=w398) -> ()  [unwired: 2 in, 2 out]
        n178 = property on="Save HPPC Report" class="Bool"("DisabledEnum"=T5."Disabled and Grayed Out" ("Disabled")) -> ()  [unwired: 2 in, 2 out]
      }
      frame "UI: Cleanup" {
        n179 = property class="VI"() -> (error out=w414:errorcluster, "FP.State"=w416:T7)  [unwired: 2 in, 1 out]
        n180 = case shown="\"Standard\", Default" w416 {
          frame "Closed" {
          }
          frame "Standard", Default {
            n181 = invoke class="VI" method="FP.Close"() -> ()  [unwired: 3 in, 3 out]
          }
        }
      }
      frame "---------- CMD ----------" {
      }
      frame "CMD: Exit" {
      }
      frame "CMD: Front Panel State" {
        n182 = Format Into String(format string="UI: Front Panel State>>%s" ("string"), w425) -> (resulting string=w424:string)  [unwired: 2 in, 1 out]
        n183 = call <vilib>:"Add State(s) to Queue__jki_lib_state_machine.vi"("State(s) in (\"\")"=w428, "State(s) at Back (\"\")"=w424) -> ("States Out"=w427:string)  [unwired: 13 in]
      }
      frame "CMD: Start Profile" {
        n184 = Unbundle By Name(w436) -> ("Profile Complete Event"=w439:refnum<user-event>, "Core.Data"=w440:variant)
        n185 = call <vilib>:"Add State(s) to Queue__jki_lib_state_machine.vi"("State(s) in Front (\"\")"="HPPC: Start Profile", "State(s) in (\"\")"=w433) -> ("States Out"=w432:string)  [unwired: 13 in]
        n186 = Variant To Data(error in=w438, type=w439, Variant=w440) -> (data=w434:refnum<user-event>, error out=w437:errorcluster)
        n187 = Bundle By Name(cluster=w436, "Profile Complete Event"=w434) -> (w435:T4)
      }
      frame "CMD: Generate Plots" {
        n188 = call <vilib>:"Add State(s) to Queue__jki_lib_state_machine.vi"("State(s) in Front (\"\")"="HPPC: Generate Plots", "State(s) in (\"\")"=w443) -> ("States Out"=w442:string)  [unwired: 13 in]
      }
      frame "CMD: Stop Profile" {
        n189 = call <vilib>:"Add State(s) to Queue__jki_lib_state_machine.vi"("State(s) in Front (\"\")"="HPPC: Stop Profile", "State(s) in (\"\")"=w447) -> ("States Out"=w446:string)  [unwired: 13 in]
      }
    }
  }
  "error out" <- w4
  "reference out" <- "reference in"
